vi "move-Motor-v2.vi"(8 "error in":errorcluster, 10 "Axis":u16(ring) items=["X", "Y", "Z"], 11 "Distance (um)":dbl) -> (0 "error out":errorcluster)   [LabVIEW 2014]
doc: "André Romero - 2023\nandretec@ifsc.usp.br\nIFSC - USP"
uses:
  Global Motors.vi
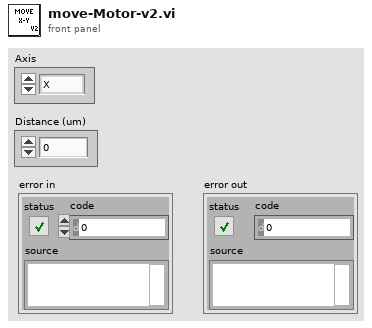
[diagram p1: front panel]
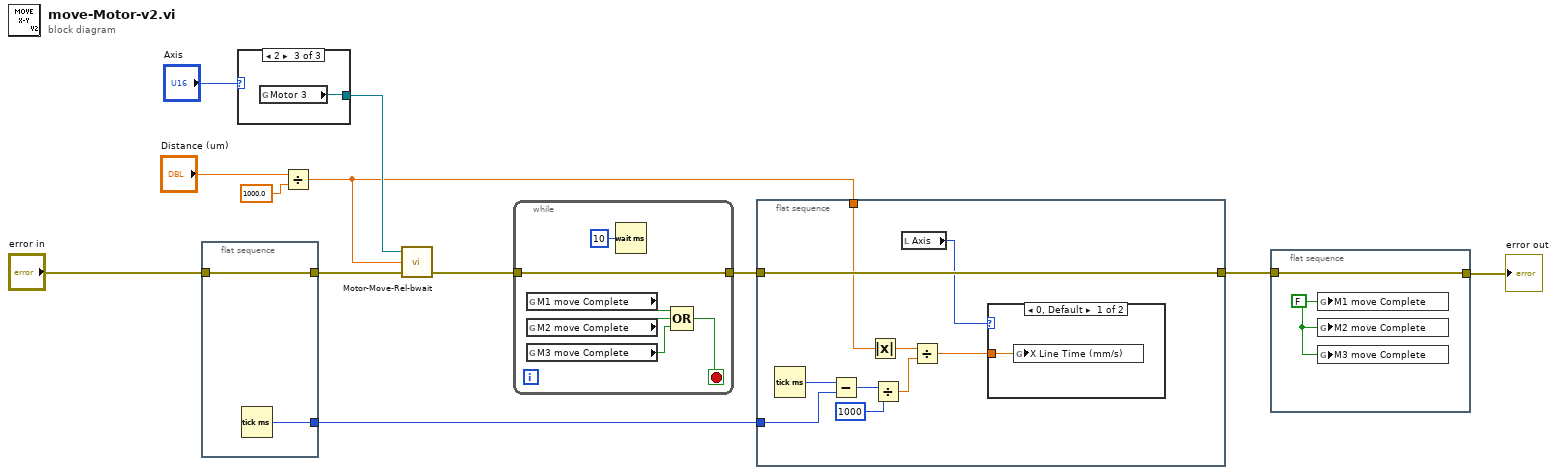
[diagram p0: block diagram]
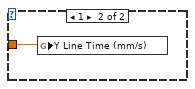
[diagram p2: hidden frame]
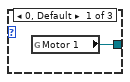
[diagram p3: hidden frame]
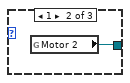
[diagram p4: hidden frame]
diagram:
  n1 = flat-sequence {
    tunnel: [w14] -> w6
    tunnel: "error in" -> [w14]
    tunnel: [w13] -> w2
    frame #0 {
      n2 = Tick Count (ms)() -> (millisecond timer value=w13:u32)
    }
  }
  n3 = case shown="2" "Axis" {
    tunnel: [w15 w16 w17] -> w12
    frame 0, Default {
      n4 = global read "Global Motors.vi" "Motor 1"() -> (w15:refnum<k7>)
    }
    frame 1 {
      n5 = global read "Global Motors.vi" "Motor 2"() -> (w16:refnum<k7>)
    }
    frame 2 {
      n6 = global read "Global Motors.vi" "Motor 3"() -> (w17:refnum<k7>)
    }
  }
  n7 = Divide(x="Distance (um)", y=1000.0 ("x")) -> (x/y=w1:dbl)
  n8 = call "Motor-Move-Rel-bwait.vi"("error"=w6, "Posição"=w1, "MG17Motor A"=w12) -> ("error out"=w9:errorcluster)  [unwired: 1 in, 1 out]
  n9 = while {
    tunnel: w9 -> [w23]
    tunnel: [w23] -> w4
    stop <- w20 stop-if-true
    n10 = global read "Global Motors.vi" "M1 move Complete"() -> (w22:bool)
    n11 = global read "Global Motors.vi" "M2 move Complete"() -> (w21:bool)
    n12 = global read "Global Motors.vi" "M3 move Complete"() -> (w18:bool)
    n13 = Wait (ms)(milliseconds to wait=u32 10) -> ()  [unwired: 1 out]
    n14 = Compound Arithmetic op=OR(w22, w21, w18) -> (w20:bool)
  }
  n15 = flat-sequence {
    tunnel: w4 -> [w33]
    tunnel: [w33] -> w3
    tunnel: w2 -> [w31]
    tunnel: w1 -> [w28]
    frame #0 {
      n16 = Tick Count (ms)() -> (millisecond timer value=w32:u32)
      n17 = Subtract(x=w32, y=w31) -> (x-y=w30:u32)
      n18 = Absolute Value(x=w28) -> (abs(x)=w26:dbl)
      n19 = Divide(x=w30, y=u32 1000) -> (x/y=w27:dbl)
      n20 = local read "Axis"() -> (w25:u16)
      n21 = Divide(x=w26, y=w27) -> (x/y=w24:dbl)
      n22 = case shown="0, Default" w25 {
        tunnel: w24 -> [w34 w35]
        frame 0, Default {
          n23 = global write "Global Motors.vi" "X Line Time (mm/s)"(w34) -> ()
        }
        frame 1 {
          n24 = global write "Global Motors.vi" "Y Line Time (mm/s)"(w35) -> ()
        }
      }
    }
  }
  n25 = flat-sequence {
    tunnel: w3 -> [w37]
    tunnel: [w37] -> w8
    frame #0 {
      w36 = FALSE ("M1 move Complete")
      n26 = global write "Global Motors.vi" "M1 move Complete"(w36) -> ()
      n27 = global write "Global Motors.vi" "M2 move Complete"(w36) -> ()
      n28 = global write "Global Motors.vi" "M3 move Complete"(w36) -> ()
    }
  }
  "error out" <- w8
